vi "Supervisor.vi"   [LabVIEW 2014, in "Supervisor.lvclass"]
uses:
  Supervisor.lvclass
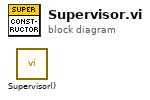
[diagram p0: block diagram]
diagram:
  n1 = call "Supervisor().vi"() -> ()  [unwired: 11 in, 1 out]
